vi "saveTimeSeries_IV.vi"(0 "1":dbl, 1 "file path (dialog if empty)":path, 2 "save?":bool, 5 "2":dbl, 7 "3":dbl, 9 "4":dbl, 11 "Error In":errorcluster, 12 "Number of Data Series":enum16{"1", "2", "3", "4"}(ring)) -> (15 "Error Out":errorcluster)   [LabVIEW 2011]
uses:
  <vilib>/Utility/file.llb/Write To Spreadsheet File (string).vi
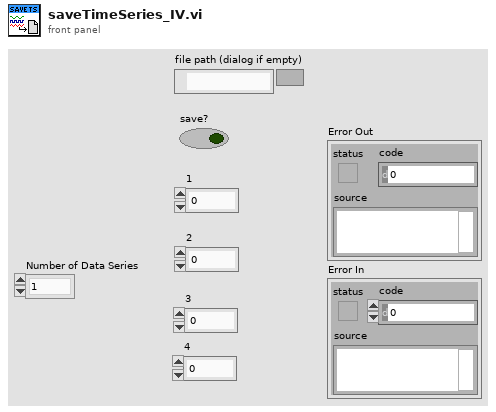
[diagram p1: front panel]
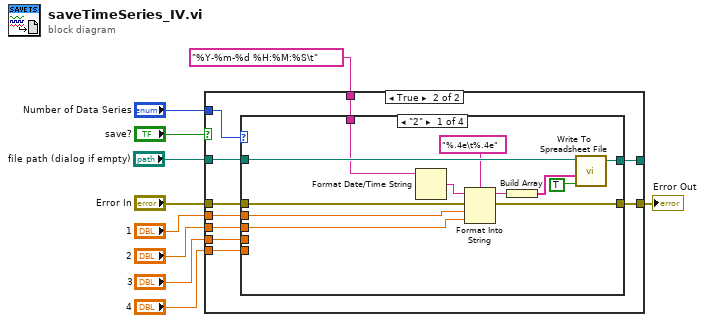
[diagram p0: block diagram]
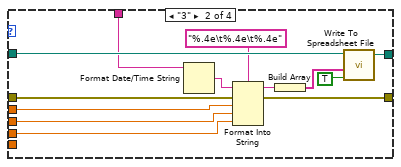
[diagram p3: hidden frame]
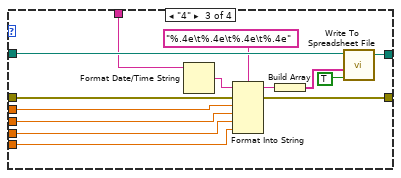
[diagram p4: hidden frame]
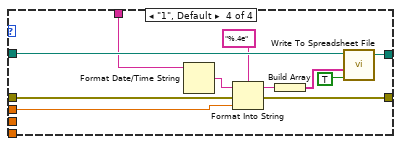
[diagram p5: hidden frame]
diagram:
  n1 = case shown="True" "save?" {
    tunnel: "3" -> [_ w22]
    tunnel: "2" -> [_ w21]
    tunnel: "1" -> [_ w20]
    tunnel: "file path (dialog if empty)" -> [w12 w19]
    tunnel: [w12 w18] -> _
    tunnel: "Error In" -> [w11 w17]
    tunnel: [w11 w16] -> w3
    tunnel: "4" -> [_ w15]
    tunnel: "Number of Data Series" -> [_ w14]
    tunnel: "%Y-%m-%d %H:%M:%S\t" ("time format string (%c)") -> [_ w13]
    frame False {
    }
    frame True {
      n2 = case shown="\"2\"" w14 {
        tunnel: w22 -> [_ w47 w61 _]
        tunnel: w21 -> [w34 w46 w60 _]
        tunnel: w20 -> [w33 w45 w59 w72]
        tunnel: w19 -> [w32 w44 w58 w71]
        tunnel: [w31 w43 w57 w70] -> w18
        tunnel: w17 -> [w26 w38 w52 w65]
        tunnel: [w25 w37 w51 w64] -> w16
        tunnel: w15 -> [_ _ w50 _]
        tunnel: w13 -> [w24 w36 w49 w63]
        frame "2" {
          n3 = Format Date/Time String(time format string (%c)=w24) -> (date/time string=w29:string)  [unwired: 2 in]
          n4 = Format Into String(format string="%.4e\t%.4e", initial string=w29, error in=w26, w33, w34) -> (resulting string=w28:string, error out=w25:errorcluster)
          n5 = Build Array(w28) -> (w27:string[])
          n6 = call-poly <vilib>:"Write To Spreadsheet File.vi"("append to file? (new file:F)"=TRUE, "1D data"=w27, "file path (dialog if empty)"=w32) -> ("new file path (Not A Path if cancelled)"=w31:path)  [unwired: 5 in]
        }
        frame "3" {
          n7 = Format Date/Time String(time format string (%c)=w36) -> (date/time string=w41:string)  [unwired: 2 in]
          n8 = Format Into String(format string="%.4e\t%.4e\t%.4e", initial string=w41, error in=w38, w45, w46, w47) -> (resulting string=w40:string, error out=w37:errorcluster)
          n9 = Build Array(w40) -> (w39:string[])
          n10 = call-poly <vilib>:"Write To Spreadsheet File.vi"("append to file? (new file:F)"=TRUE, "1D data"=w39, "file path (dialog if empty)"=w44) -> ("new file path (Not A Path if cancelled)"=w43:path)  [unwired: 5 in]
        }
        frame "4" {
          n11 = Format Date/Time String(time format string (%c)=w49) -> (date/time string=w55:string)  [unwired: 2 in]
          n12 = Format Into String(format string="%.4e\t%.4e\t%.4e\t%.4e", initial string=w55, error in=w52, w59, w60, w61, w50) -> (resulting string=w54:string, error out=w51:errorcluster)
          n13 = Build Array(w54) -> (w53:string[])
          n14 = call-poly <vilib>:"Write To Spreadsheet File.vi"("append to file? (new file:F)"=TRUE, "1D data"=w53, "file path (dialog if empty)"=w58) -> ("new file path (Not A Path if cancelled)"=w57:path)  [unwired: 5 in]
        }
        frame "1", Default {
          n15 = Format Date/Time String(time format string (%c)=w63) -> (date/time string=w68:string)  [unwired: 2 in]
          n16 = Format Into String(format string="%.4e", initial string=w68, error in=w65, w72) -> (resulting string=w67:string, error out=w64:errorcluster)
          n17 = Build Array(w67) -> (w66:string[])
          n18 = call-poly <vilib>:"Write To Spreadsheet File.vi"("append to file? (new file:F)"=TRUE, "1D data"=w66, "file path (dialog if empty)"=w71) -> ("new file path (Not A Path if cancelled)"=w70:path)  [unwired: 5 in]
        }
      }
    }
  }
  "Error Out" <- w3
